vi "withlocalvariables.vi"() -> ()   [LabVIEW 2013]
panel:
  out "Task 2":dbl(slide) scale=0.0..10.0
  out "Task 1":dbl(slide) scale=0.0..10.0
  in  "stop":bool
  out "Numeric":dbl
  in  "OK Button":bool
  in  "Tank":dbl(slide) scale=0.0..10.0
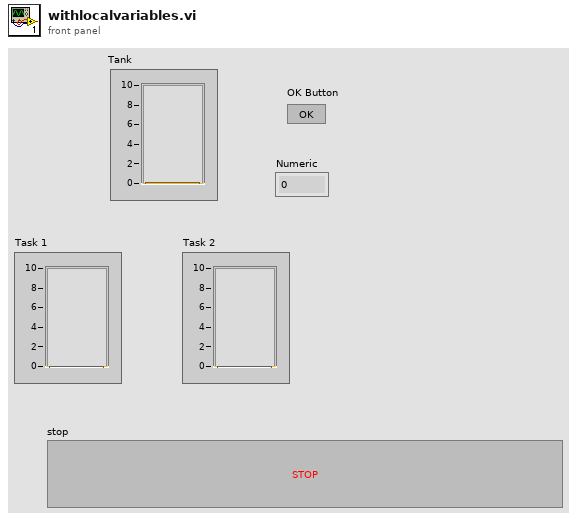
[diagram p1: front panel]
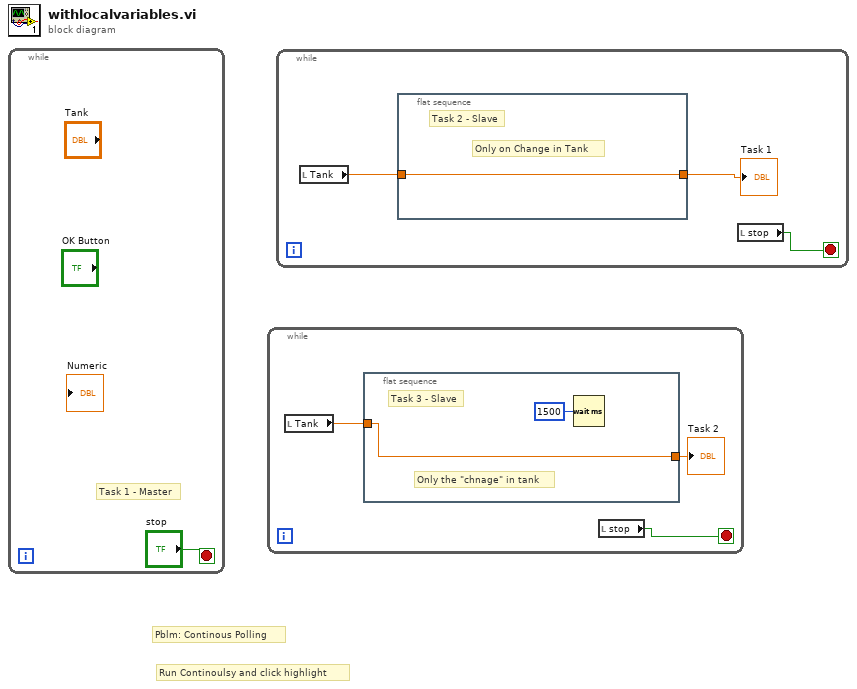
[diagram p0: block diagram]
diagram:
  # "Run Continoulsy and click highlight"
  # "Pblm: Continous Polling"
  n1 = while {
    stop <- "stop" stop-if-true
    # "Task 1 - Master"
  }
  n2 = while {
    stop <- w2 stop-if-true
    n3 = local read "Tank"() -> (w4:dbl)
    n4 = flat-sequence {
      tunnel: w4 -> [w6]
      tunnel: [w6] -> w3
      frame #0 {
        # "Only the \"chnage\" in tank"
        # "Task 3 - Slave"
        n5 = Wait (ms)(milliseconds to wait=u32 1500) -> ()  [unwired: 1 out]
      }
    }
    n6 = local read "stop"() -> (w2:bool)
    "Task 2" <- w3
  }
  n7 = while {
    stop <- w7 stop-if-true
    n8 = local read "Tank"() -> (w9:dbl)
    n9 = flat-sequence {
      tunnel: w9 -> [w10]
      tunnel: [w10] -> w8
      frame #0 {
        # "Only on Change in Tank"
        # "Task 2 - Slave"
      }
    }
    n10 = local read "stop"() -> (w7:bool)
    "Task 1" <- w8
  }
